vi "Close comm handler.vi"(8 "error in (no error)":errorcluster, 11 "WAMP Client in":refnum<class "WAMP Client.lvclass">) -> (0 "error out":errorcluster, 3 "WAMP Client out":refnum<class "WAMP Client.lvclass">)   [LabVIEW 2020, in "wamplv.lvlib" / "WAMP Client.lvclass"]
uses:
  WAMP Client.lvclass
  WAMP Client.lvclass/WAMP Client.ctl
  Private/Comm Handlers/ICommHandler/ICommHandler.lvclass
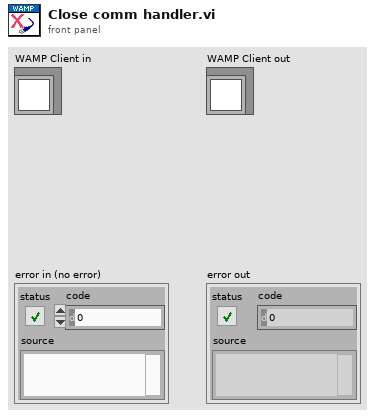
[diagram p1: front panel]
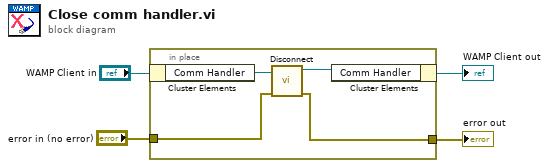
[diagram p0: block diagram]
diagram:
  n1 = in-place {
    in-place-border: "error in (no error)" -> [w6]
    in-place-border: [w5] -> w1
    n2 = in-place-cluster #1("WAMP Client in") -> ("Comm Handler"=w8:refnum<class "ICommHandler.lvclass">)
    n3 = call-dynamic "Disconnect.vi"("error in (no error)"=w6, "ICommHandler in"=w8) -> ("error out"=w5:errorcluster, "ICommHandler out"=w7:refnum<class "ICommHandler.lvclass">)  [unwired: 8 in]
    n4 = in-place-cluster #1("Comm Handler"=w7) -> (→"WAMP Client out":refnum<class "WAMP Client.lvclass">)
  }
  "error out" <- w1
